vi "Wrap.vi"(11 "gesture":refnum<class "Gesture.lvclass">) -> (3 "Gesture Wrapper":refnum<class "Gesture Wrapper.lvclass">)   [LabVIEW 2019, in "Gesture Wrapper.lvclass"]
doc: "Wrap the gesture in a Gesture Wrapper object."
uses:
  Gesture Wrapper.lvclass
  Gesture/Gesture.lvclass
  Gesture Wrapper.lvclass/Gesture Wrapper.ctl
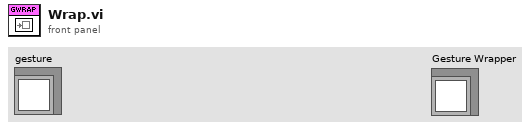
[diagram p1: front panel]
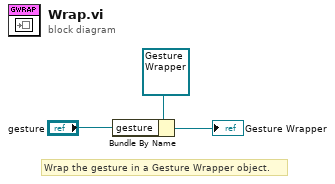
[diagram p0: block diagram]
diagram:
  # "Wrap the gesture in a Gesture Wrapper object."
  n1 = Bundle By Name(cluster=refnum<class "Gesture Wrapper.lvclass"> refnum ("Gesture Wrapper"), "gesture"="gesture") -> (→"Gesture Wrapper":refnum<class "Gesture Wrapper.lvclass">)
